vi "Init.vi"(8 "error in (no error)":errorcluster, 10 "ICameraTestingUI":refnum<class "ICameraTestingUI.lvclass">, 11 "CameraTesting in":refnum<class "CameraTesting.lvclass">) -> (0 "error out":errorcluster, 3 "CameraTesting out":refnum<class "CameraTesting.lvclass">)   [LabVIEW 2020, in "CameraTesting.lvlib" / "CameraTesting.lvclass"]
uses:
  CameraTesting.lvclass
  C:/Program Files (x86)/National Instruments/LabVIEW 2020/vi.lib/ActorFramework/Actor/Actor.lvclass
  ICameraTestingUI/ICameraTestingUI/ICameraTestingUI.lvclass
  Private/TypeDef/MsgInitStates.ctl
  CameraTesting.lvclass/CameraTesting.ctl
  <vilib>/ActorFramework/Actor/Actor.lvclass
  ICameraTestingUI/ICameraTestingUI Messages/ShowFP Msg/ShowFP Msg.lvclass/ShowFP Msg.ctl
  <vilib>/ActorFramework/Message Enqueuer/Message Enqueuer.lvclass/Message Enqueuer.ctl
  <vilib>/ActorFramework/Message Enqueuer/Enqueue.vi
  ICameraTestingUI/ICameraTestingUI Messages/ShowFP Msg/ShowFP Msg.lvclass
  C:/Program Files (x86)/National Instruments/LabVIEW 2020/vi.lib/ActorFramework/Message/Message.lvclass
  <vilib>/ActorFramework/Message Priority Queue/Priority Enqueue.vi
  Camera/ICamera/ICamera/ICamera.lvclass
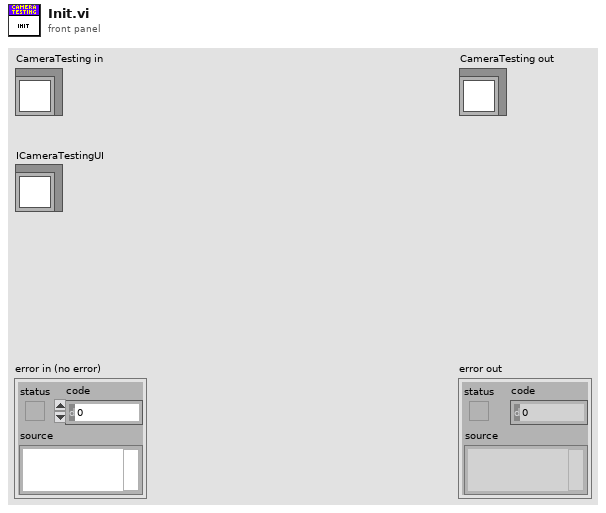
[diagram p1: front panel]
types:
  T1 = typedef "CameraTesting.lvlib/CameraTesting.lvclass/MsgInitStates.ctl" = enum16{"Create Events", "Inizialize Camera", "Camera Events Request", "Enumeration Camera Video Options", "Events Registration", "Launch User Interface", "Show UI"}
  T2 = typedef "ICamera.lvlib/ICamera.lvclass/Events.ctl" = cluster{"CameraStreamDataUpdate":T3}
  T3 = typedef "ICamera.lvlib/ICamera.lvclass/StreamDataEvent.ctl" = refnum<user-event>
  T4 = typedef "ICamera.lvlib/ICamera.lvclass/VideoOptionsCodes.ctl" = cluster{"FrameRateCodesList":cluster{"Description":string, "Code":u8}[], "VideoResolutionCodesList":cluster{"Description":string, "Code":u8}[], "ImageTypeCodesList":cluster{"Description":string, "Code":u8}[]}
  T5 = typedef "CameraTesting.lvlib/CameraTesting.lvclass/PrivateEvents.ctl" = cluster{"ActorStopped":T6}
  T6 = typedef "CameraTesting.lvlib/CameraTesting.lvclass/ActorStopped.ctl" = refnum<user-event>
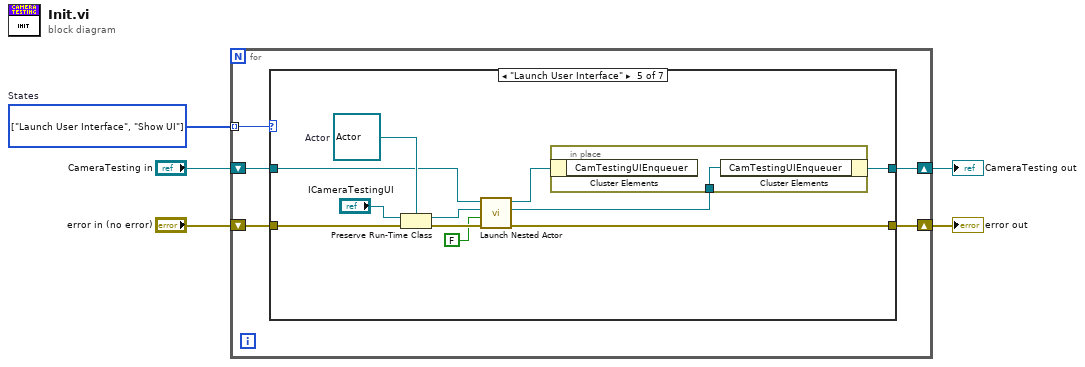
[diagram p0: block diagram]
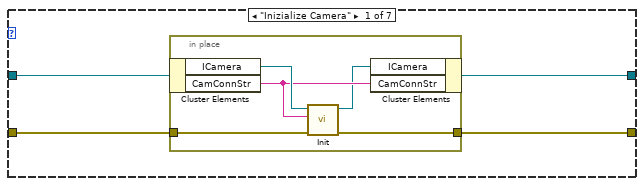
[diagram p2: hidden frame]
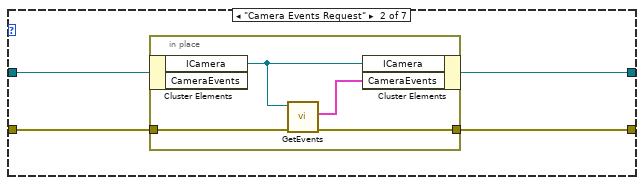
[diagram p3: hidden frame]
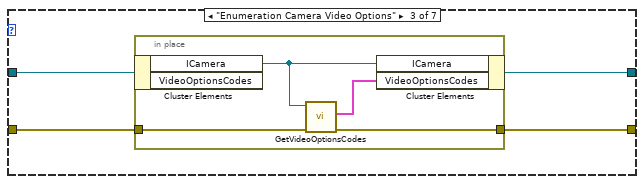
[diagram p4: hidden frame]
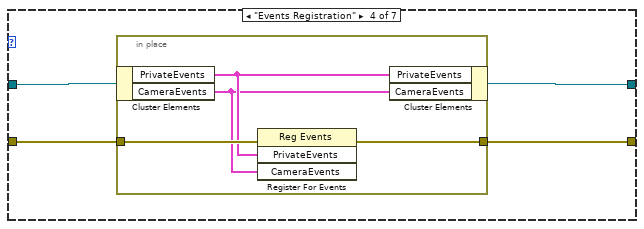
[diagram p5: hidden frame]
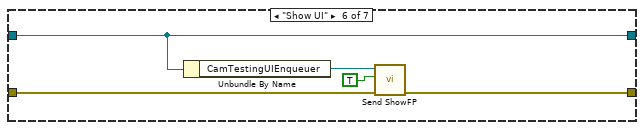
[diagram p6: hidden frame]
diagram:
  w5 = T1[] [enum."Launch User Interface", enum."Show UI"] items=["Create Events", "Inizialize Camera", "Camera Events Request", "Enumeration Camera Video Options", "Events Registration", "Launch User Interface", "Show UI"]  # States
  n1 = for {
    tunnel: w5 -> [w10] mode=indexing
    shift-right: [w6] -> w2
    shift-left: "CameraTesting in" -> [w9]
    shift-right: [w7] -> w1
    shift-left: "error in (no error)" -> [w8]
    n2 = case shown="\"Launch User Interface\"" w10 {
      tunnel: w9 -> [w14 w23 w31 w39 w48 w60 w62]
      tunnel: w8 -> [w13 w22 w30 w38 w49 w58 w61]
      tunnel: [w12 w21 w29 w37 w47 w57 w61] -> w7
      tunnel: [w11 w20 w28 w36 w45 w60 w62] -> w6
      frame "Inizialize Camera" {
        n3 = in-place {
          in-place-border: w13 -> [w16]
          in-place-border: [w15] -> w12
          n4 = in-place-cluster #1(w14) -> ("ICamera"=w19:refnum<class "ICamera.lvclass">, "CamConnStr"=w18:string)
          n5 = call-dynamic "Init.vi"("error in (no error)"=w16, "Connection String"=w18, "ICamera in"=w19) -> ("error out"=w15:errorcluster, "ICamera out"=w17:refnum<class "ICamera.lvclass">)  [unwired: 7 in]
          n6 = in-place-cluster #1("ICamera"=w17, "CamConnStr"=w18) -> (w11:refnum<class "CameraTesting.lvclass">)
        }
      }
      frame "Camera Events Request" {
        n7 = in-place {
          in-place-border: w22 -> [w25]
          in-place-border: [w24] -> w21
          n8 = in-place-cluster #2(w23) -> ("ICamera"=w27:refnum<class "ICamera.lvclass">)  [unwired: 1 out]
          n9 = call-dynamic "GetEvents.vi"("error in (no error)"=w25, "ICamera in"=w27) -> ("error out"=w24:errorcluster, "CameraEvents"=w26:T2)  [unwired: 7 in, 1 out]
          n10 = in-place-cluster #2("ICamera"=w27, "CameraEvents"=w26) -> (w20:refnum<class "CameraTesting.lvclass">)
        }
      }
      frame "Enumeration Camera Video Options" {
        n11 = in-place {
          in-place-border: w30 -> [w35]
          in-place-border: [w34] -> w29
          n12 = in-place-cluster #3(w31) -> ("ICamera"=w33:refnum<class "ICamera.lvclass">)  [unwired: 1 out]
          n13 = call-dynamic "GetVideoOptionsCodes.vi"("error in (no error)"=w35, "ICamera in"=w33) -> ("error out"=w34:errorcluster, "VideoOptionsCodes"=w32:T4)  [unwired: 7 in, 1 out]
          n14 = in-place-cluster #3("ICamera"=w33, "VideoOptionsCodes"=w32) -> (w28:refnum<class "CameraTesting.lvclass">)
        }
      }
      frame "Events Registration" {
        n15 = in-place {
          in-place-border: w38 -> [w43]
          in-place-border: [w42] -> w37
          n16 = in-place-cluster #4(w39) -> ("PrivateEvents"=w41:T5, "CameraEvents"=w40:T2)
          n17 = register-events(error in=w43, w41, w40) -> (error out=w42:errorcluster)  [unwired: 1 in, 1 out]
          n18 = in-place-cluster #4("PrivateEvents"=w41, "CameraEvents"=w40) -> (w36:refnum<class "CameraTesting.lvclass">)
        }
      }
      frame "Launch User Interface" {
        w50 = refnum<class "Actor.lvclass"> refnum  # Actor
        n19 = Preserve Run-Time Class(object in="ICameraTestingUI", error in=w49, 2:w50) -> (object out=w53:refnum<class "Actor.lvclass">, error out=w54:errorcluster)
        n20 = call <vilib>:"Launch Nested Actor.vi"("error in (no error)"=w54, "Auto-stop? (T)"=FALSE, "Nested Actor"=w53, "Caller Actor in"=w48) -> ("error out"=w47:errorcluster, "Nested Actor's Enqueuer"=w44:refnum<class "Message Enqueuer.lvclass">, "Caller Actor out"=w46:refnum<class "CameraTesting.lvclass">)  [unwired: 5 in]
        n21 = in-place {
          in-place-border: w44 -> [w55]
          n22 = in-place-cluster #5(w46) -> ()  [unwired: 1 out]
          n23 = in-place-cluster #5("CamTestingUIEnqueuer"=w55) -> (w45:refnum<class "CameraTesting.lvclass">)
        }
      }
      frame "Show UI" {
        n24 = Unbundle By Name(w60) -> ("CamTestingUIEnqueuer"=w59:refnum<class "Message Enqueuer.lvclass">)
        n25 = call "Send ShowFP.vi"("error in (no error)"=w58, "ResetFP"=TRUE, "Message Enqueuer"=w59) -> ("error out"=w57:errorcluster)  [unwired: 7 in, 1 out]
      }
      frame "Create Events" {
      }
    }
  }
  "error out" <- w1
  "CameraTesting out" <- w2
